vi "多参数质控参数设置.vi"(11 "质控参数设置":T1) -> (3 "输出簇":T2)   [LabVIEW 2016, in "斯坦道多参数.lvlib"]
uses:
  <vilib>/Utility/miscctls.llb/LVPointTypeDef.ctl
panel:
  in  "浊度标准液标准浓度":dbl
  in  "电导率标准液标准浓度":dbl
  in  "溶解氧标准液标准浓度":dbl
  in  "酸碱度标准液标准浓度":dbl
  in  "取消":bool
  in  "确定":bool
  in  "水温标准液标准浓度":dbl
  # "质控参数设置"
  # "监测参数"
  # "水温"
  # "酸碱度"
  # "溶解氧"
  # "电导率"
  # "浊度"
  # "标样核查标准液浓度"
  # "质控参数设置"
  # "监测参数"
  # "水温"
  # "酸碱度"
  # "溶解氧"
  # "电导率"
  # "浊度"
  # "标样核查标准液浓度"
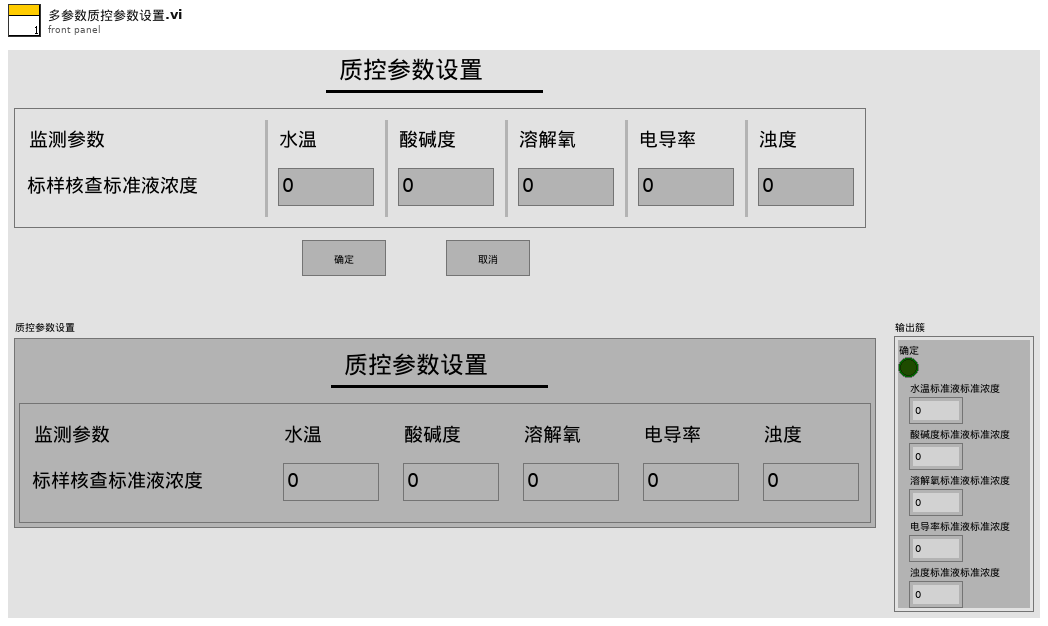
[diagram p1: front panel]
types:
  T1 = cluster{"水温标准液标准浓度":dbl, "酸碱度标准液标准浓度":dbl, "溶解氧标准液标准浓度":dbl, "电导率标准液标准浓度":dbl, "浊度标准液标准浓度":dbl}
  T2 = cluster{"确定":bool, "水温标准液标准浓度":dbl, "酸碱度标准液标准浓度":dbl, "溶解氧标准液标准浓度":dbl, "电导率标准液标准浓度":dbl, "浊度标准液标准浓度":dbl}
  T3 = typedef "LVPointTypeDef.ctl" = cluster{"Horizontal":i16, "Vertical":i16}
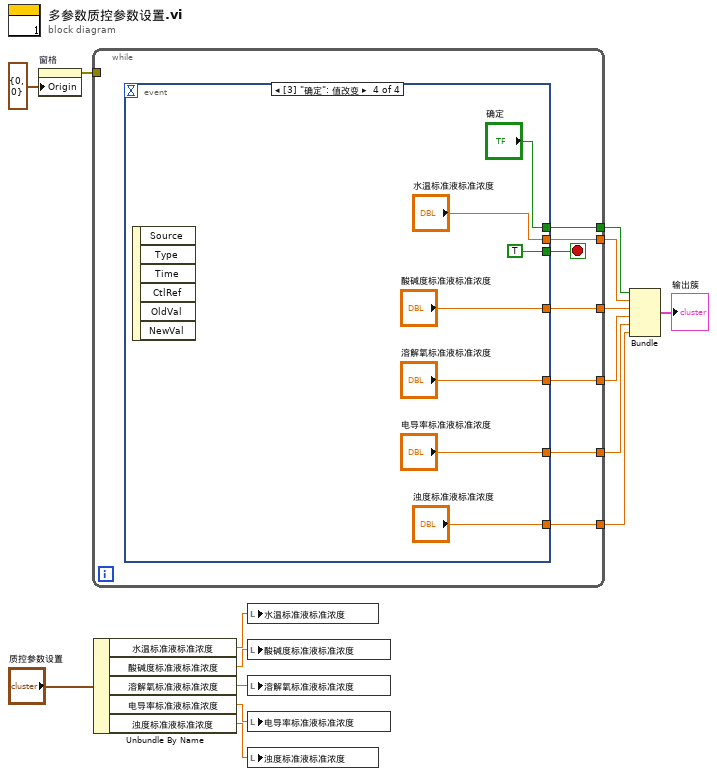
[diagram p0: block diagram]
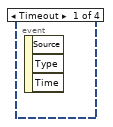
[diagram p2: hidden frame]
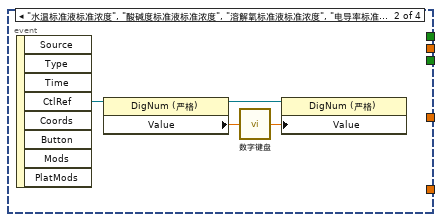
[diagram p3: hidden frame]
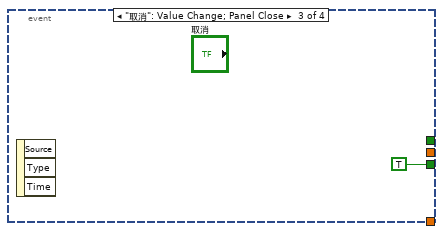
[diagram p4: hidden frame]
diagram:
  n1 = property on="窗格" class="Pane"("Origin"=T3 {"Horizontal"=0, "Vertical"=0} ("原点")) -> (error out=w14:errorcluster)  [unwired: 2 in, 1 out]
  n2 = while {
    tunnel: w14 -> [_]
    tunnel: [w21] -> w13
    tunnel: [w20] -> w12
    tunnel: [w19] -> w11
    tunnel: [w18] -> w10
    tunnel: [w17] -> w9
    tunnel: [w16] -> w3
    stop <- w22 stop-if-true
    n3 = event shown="[3] \"确定\": 值改变" {
      selector: _ -> [_ _ _ _]
      dyn-events: _ -> [_ _ _ _]
      timeout: _ -> [_ _ _ _]
      tunnel: [_ _ TRUE TRUE] -> w22
      tunnel: [_ _ _ "水温标准液标准浓度"] -> w21
      tunnel: [_ _ _ "酸碱度标准液标准浓度"] -> w20
      tunnel: [_ _ _ "溶解氧标准液标准浓度"] -> w19
      tunnel: [_ _ _ "电导率标准液标准浓度"] -> w18
      tunnel: [_ _ _ "确定"] -> w17
      tunnel: [_ _ _ "浊度标准液标准浓度"] -> w16
      event Timeout {
        n4 = event-data() -> ()  [unwired: 1 in, 3 out]
      }
      event "水温标准液标准浓度", "酸碱度标准液标准浓度", "溶解氧标准液标准浓度", "电导率标准液标准浓度", "浊度标准液标准浓度": Mouse Down {
        n5 = event-data() -> ("CtlRef"=w26:refnum<vi>)  [unwired: 1 in, 7 out]
        n6 = property class="DigNum (严格)"(reference=w26) -> (reference out=w25:refnum<vi>, "Value"=w24:dbl)  [unwired: 1 in, 1 out]
        n7 = call "数字键盘.vi"("OldNumber"=w24) -> ("NewNumber"=w23:dbl)
        n8 = property class="DigNum (严格)"(reference=w25, "Value"=w23) -> ()  [unwired: 1 in, 2 out]
      }
      event "取消": Value Change; Panel Close {
        n9 = event-data() -> ()  [unwired: 1 in, 3 out]
      }
      event "确定": Value Change {
        n10 = event-data() -> ()  [unwired: 1 in, 6 out]
      }
    }
  }
  n11 = Unbundle By Name("质控参数设置") -> ("水温标准液标准浓度"=w8:dbl, "酸碱度标准液标准浓度"=w5:dbl, "溶解氧标准液标准浓度"=w6:dbl, "电导率标准液标准浓度"=w7:dbl, "浊度标准液标准浓度"=w4:dbl)
  n12 = local write "水温标准液标准浓度"(w8) -> ()
  n13 = local write "酸碱度标准液标准浓度"(w5) -> ()
  n14 = local write "溶解氧标准液标准浓度"(w6) -> ()
  n15 = local write "电导率标准液标准浓度"(w7) -> ()
  n16 = local write "浊度标准液标准浓度"(w4) -> ()
  n17 = Bundle("确定"=w9, "水温标准液标准浓度"=w13, "酸碱度标准液标准浓度"=w12, "溶解氧标准液标准浓度"=w11, "电导率标准液标准浓度"=w10, "浊度标准液标准浓度"=w3) -> (→"输出簇":T2)  [unwired: 1 in]
